vi "POI Autogen number entry window.vi"() -> (0 "Cancelled":bool, 2 "Number of POI":i32)   [LabVIEW 2013]
panel:
  in  "Points":i32=30 min=3 max=100
  in  "Cancel":bool
  in  "Proceed":bool
  # "Enter the number of points of interest to generate automatically."
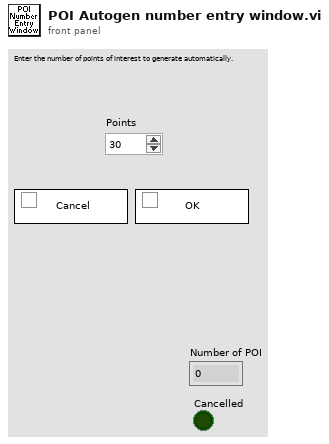
[diagram p1: front panel]
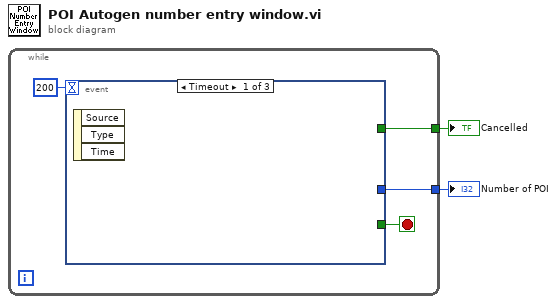
[diagram p0: block diagram]
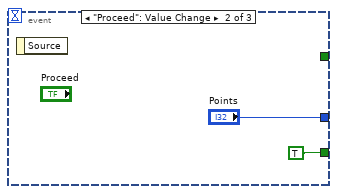
[diagram p2: hidden frame]
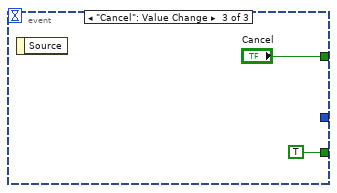
[diagram p3: hidden frame]
diagram:
  n1 = while {
    tunnel: [w5] -> w2
    tunnel: [w4] -> w1
    stop <- w6 stop-if-true
    n2 = event shown="[0] Timeout" {
      selector: _ -> [_ _ _]
      dyn-events: _ -> [_ _ _]
      timeout: 200 -> [_ _ _]
      tunnel: [_ TRUE TRUE] -> w6
      tunnel: [_ _ "Cancel"] -> w5
      tunnel: [_ "Points" _] -> w4
      event Timeout {
        n3 = event-data() -> ()  [unwired: 1 in, 3 out]
      }
      event "Proceed": Value Change {
        n4 = event-data() -> ()  [unwired: 1 in, 1 out]
      }
      event "Cancel": Value Change {
        n5 = event-data() -> ()  [unwired: 1 in, 1 out]
      }
    }
  }
  "Cancelled" <- w2
  "Number of POI" <- w1
